vi "InitDrv.vi"() -> (0 "Boards":u8)   [LabVIEW 2015]
uses:
  ESLSCDLL.dll
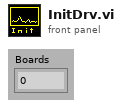
[diagram p1: front panel]
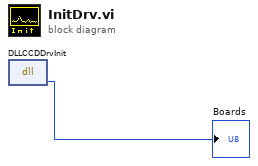
[diagram p0: block diagram]
diagram:
  n1 = dll-call lib="C:/ENTW/PCIE/64bit/lv64/2camx/board.vis/ESLSCDLL.dll" fn="DLLCCDDrvInit"() -> ("Rückgabetyp"=→"Boards":u8)  [unwired: 3 in, 2 out]
